vi "JSONtext Clusters to Objects or Arrays.vi"() -> ()   [LabVIEW 2013]
uses:
  JSONtext.lvlib
panel:
  out "<JSON> Array":string
  out "<JSON> Object":string
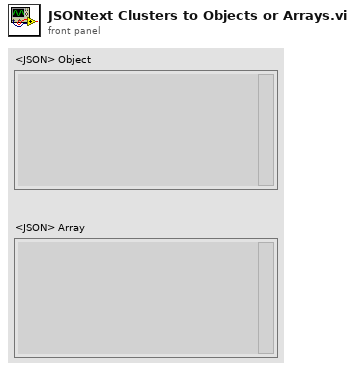
[diagram p1: front panel]
types:
  T1 = cluster{"MyString":string, "MyNum":dbl, "<JSON>MyJSON":string}
  T2 = cluster{string, "MyNum":dbl, "<JSON>MyJSON":string}
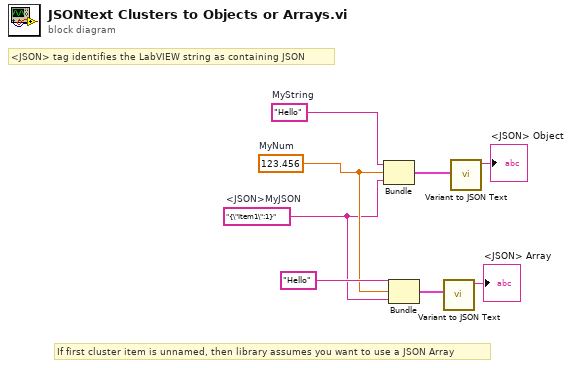
[diagram p0: block diagram]
diagram:
  w3 = "{\"Item1\":1}"  # <JSON>MyJSON
  w4 = 123.456  # MyNum
  w8 = "Hello"  # MyString
  # "<JSON> tag identifies the LabVIEW string as containing JSON"
  # "If first cluster item is unnamed, then library assumes you want to use a JSON Array"
  n1 = Bundle("MyString"=w8, "MyNum"=w4, "<JSON>MyJSON"=w3) -> (w7:T1)  [unwired: 1 in]
  n2 = Bundle("Hello", "MyNum"=w4, "<JSON>MyJSON"=w3) -> (w1:T2)  [unwired: 1 in]
  n3 = call "Variant to JSON Text.vi"("Variant"=w1) -> ("<JSON>"=→"<JSON> Array":string)  [unwired: 9 in, 1 out]
  n4 = call "Variant to JSON Text.vi"("Variant"=w7) -> ("<JSON>"=→"<JSON> Object":string)  [unwired: 9 in, 1 out]
